vi "sub_qam_symbol_map_gen.vi"(9 "Gray code?":bool, 11 "M-QAM":i32) -> (3 "symbol map":cdb[](array[numeric]))   [LabVIEW 2014]
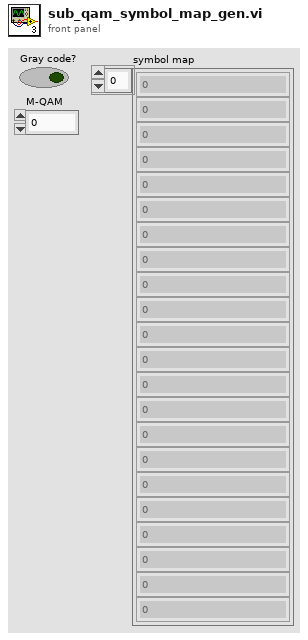
[diagram p1: front panel]
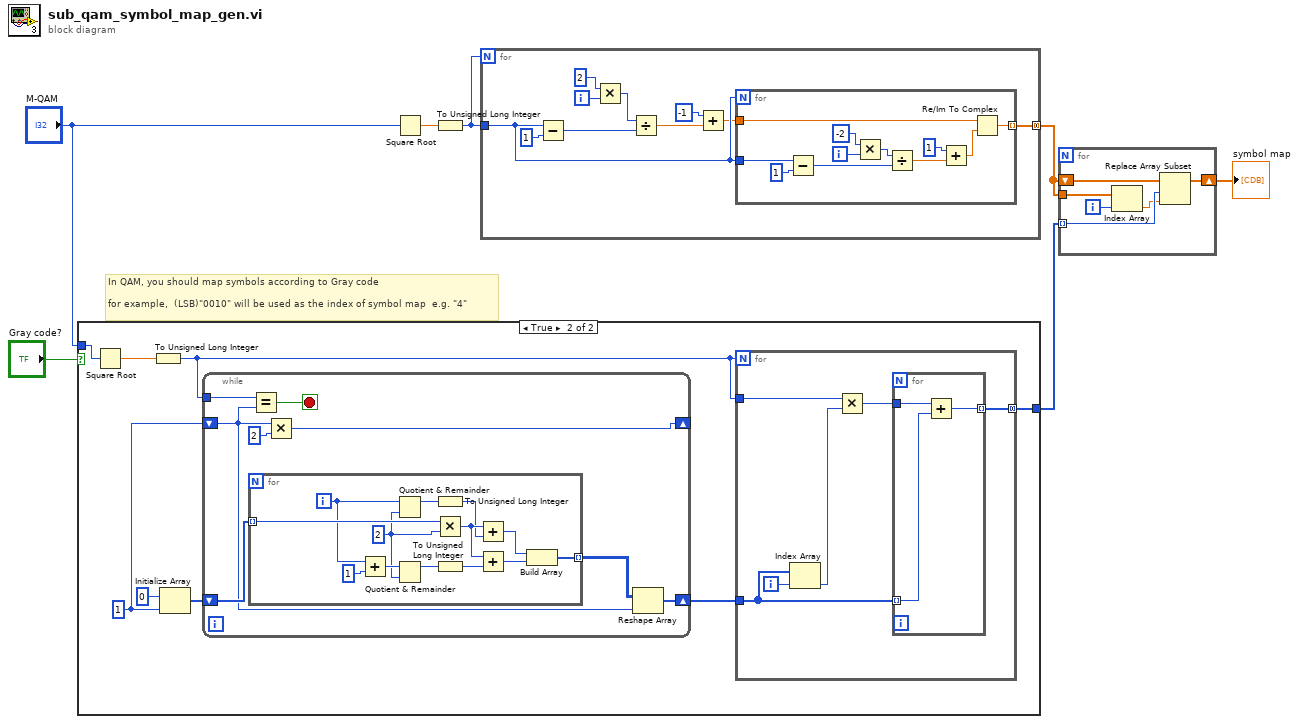
[diagram p0: block diagram]
diagram:
  # "In QAM, you should map symbols according to Gray code\n\nfor example,  (LSB)\"0010\" will be used as the index of symbol map  e.g. \"4\""
  n1 = case shown="True" "Gray code?" {
    tunnel: "M-QAM" -> [w9 w14]
    tunnel: [w8 w11] -> w3
    frame False {
      n2 = for {
        N: w9 -> [_]
        tunnel: [w10] -> w8 mode=indexing
        i -> [w10]
      }
    }
    frame True {
      w16 = u32 1
      n3 = Square Root(x=w14) -> (sqrt(x)=w15:dbl)
      n4 = To Unsigned Long Integer(number=w15) -> (unsigned 32bit integer=w12:u32)
      n5 = Initialize Array(u32 0, w16) -> (w17:u32[])
      n6 = while {
        tunnel: w12 -> [w33]
        shift-right: [w35] -> _
        shift-left: w16 -> [w29]
        shift-right: [w28] -> w13
        shift-left: w17 -> [w31]
        stop <- w32 stop-if-true
        n7 = for {
          tunnel: w31 -> [w48] mode=indexing
          tunnel: [w38] -> w30 mode=indexing
          i -> [w47]
          w44 = u32 2
          n8 = Add(x=w47, y=u32 1) -> (x+y=w45:u32)
          n9 = Quotient & Remainder(x=w47, y=w44) -> (x-y*floor(x/y)=w37:u32)  [unwired: 1 out]
          n10 = Quotient & Remainder(x=w45, y=w44) -> (x-y*floor(x/y)=w36:u32)  [unwired: 1 out]
          n11 = To Unsigned Long Integer(number=w37) -> (unsigned 32bit integer=w40:u32)
          n12 = Multiply(x=w48, y=w44) -> (x*y=w41:u32)
          n13 = To Unsigned Long Integer(number=w36) -> (unsigned 32bit integer=w39:u32)
          n14 = Add(x=w41, y=w40) -> (x+y=w43:u32)
          n15 = Add(x=w41, y=w39) -> (x+y=w42:u32)
          n16 = Build Array(w43, w42) -> (w38:u32[])
        }
        n17 = Equal?(x=w33, y=w29) -> (x = y?=w32:bool)
        n18 = Multiply(x=w29, y=u32 2) -> (x*y=w35:u32)
        n19 = Reshape Array(w30, w29) -> (w28:u32[])
      }
      n20 = for {
        N: w12 -> [_]
        tunnel: w13 -> [w21]
        tunnel: w12 -> [w22]
        tunnel: [w19] -> w11 mode=concatenating
        i -> [w24]
        n21 = Index Array(array=w21, index=w24) -> (element=w23:u32)
        n22 = Multiply(x=w22, y=w23) -> (x*y=w20:u32)
        n23 = for {
          tunnel: w21 -> [w26] mode=indexing
          tunnel: w20 -> [w27]
          tunnel: [w25] -> w19 mode=indexing
          n24 = Add(x=w27, y=w26) -> (x+y=w25:u32)
        }
      }
    }
  }
  n25 = Square Root(x="M-QAM") -> (sqrt(x)=w6:dbl)
  n26 = To Unsigned Long Integer(number=w6) -> (unsigned 32bit integer=w5:u32)
  n27 = for {
    N: w5 -> [_]
    tunnel: w5 -> [w51]
    tunnel: [w49] -> w2 mode=concatenating
    i -> [w56]
    n28 = Subtract(x=w51, y=u32 1) -> (x-y=w54:u32)
    n29 = Multiply(x=u32 2, y=w56) -> (x*y=w55:u32)
    n30 = Divide(x=w55, y=w54) -> (x/y=w53:dbl)
    n31 = Add(x=-1, y=w53) -> (x+y=w50:dbl)
    n32 = for {
      N: w51 -> [_]
      tunnel: w51 -> [w65]
      tunnel: w50 -> [w61]
      tunnel: [w59] -> w49 mode=indexing
      i -> [w63]
      n33 = Subtract(x=w65, y=u32 1) -> (x-y=w68:u32)
      n34 = Multiply(x=-2, y=w63) -> (x*y=w69:i32)
      n35 = Divide(x=w69, y=w68) -> (x/y=w67:dbl)
      n36 = Add(x=1, y=w67) -> (x+y=w60:dbl)
      n37 = Re/Im To Complex(1:w60, 2:w61) -> (0:w59:cdb)
    }
  }
  n38 = for {
    tunnel: w2 -> [w75]
    tunnel: w3 -> [w72] mode=indexing
    shift-right: [w73] -> w1
    shift-left: w2 -> [w74]
    i -> [w71]
    n39 = Index Array(array=w75, index=w71) -> (element=w70:cdb)
    n40 = Replace Array Subset(array=w74, new element=w70, index=w72) -> (w73:cdb[])
  }
  "symbol map" <- w1
